vi "Convert to KRobot.vi"(10 "scale":dbl=1.0, 11 "Graphical Elements In":T2[](array[typedef])) -> (0 "Array":dbl[][][](array[numeric]) format="%#_3g", 2 "Kinematic Robot":refnum<class "NI_Robotics_Serial Robot Arm.lvclass">, 3 "Graphical Elements In 2":T2[](array[typedef]))   [LabVIEW 2017, in "NI_Robotics_3DKinematics.lvlib"]
uses:
  <vilib>/robotics/Kinematics/Plotting/NI_Robotics_3DKinematics.lvlib
  <vilib>/robotics/Kinematics/Robot/NI_Robotics_Serial Robot Arm.lvclass
  <vilib>/robotics/Kinematics/Plotting/Tree Element.ctl
  <vilib>/robotics/Kinematics/Plotting/Element Type.ctl
  <vilib>/robotics/Kinematics/Plotting/Joint Type.ctl
  <vilib>/Analysis/Matrix/Datatypes/RealMatrix.ctl
  <vilib>/robotics/Kinematics/Link/Joint Type.ctl
  <vilib>/robotics/Kinematics/Link/NI_Robotics_Link.lvclass
  <vilib>/Analysis/_algsub.llb/Real Vector Norm.vi
  <vilib>/Analysis/baseanly.llb/Real A x B.vi
  <vilib>/Analysis/baseanly.llb/Outer Product.vi
  <vilib>/Analysis/baseanly.llb/Real Outer Product.vi
  <vilib>/robotics/Kinematics/Create Lie Group Matrix.vi
  <vilib>/Analysis/Matrix/Numeric/Conversions/Array To Matrix - RA2.vi
  <vilib>/Analysis/7linalg.llb/Solve Linear Equations (multiple right hand).vi
  <vilib>/Analysis/Matrix/Numeric/Add/Add.vi
  <vilib>/Analysis/Matrix/Numeric/Add/Add - RM,RM.vi
  <vilib>/Analysis/Matrix/Numeric/Multiply/Multiply.vi
  <vilib>/Analysis/Matrix/Numeric/Multiply/Multiply - R,RM.vi
  <vilib>/Analysis/Matrix/Numeric/Multiply/Multiply - RM,R.vi
  <vilib>/Analysis/7linalg.llb/Create Special Matrix.vi
  <vilib>/Analysis/7linalg.llb/Create Special Real Matrix.vi
  <vilib>/Utility/AngleManip/Degrees to Radians (Scalar DBL).vi
  <vilib>/robotics/Kinematics/NI_Kinematics.lvlib
  <vilib>/Analysis/Matrix/NI_Matrix.lvlib
  <vilib>/Analysis/NI_AALPro.lvlib
  <vilib>/Analysis/NI_AALBase.lvlib
  <vilib>/Utility/AngleManip/NI_AngleManipulation.lvlib
panel:
  out "Array 3":T1[](array[typedef])
  out "A x B":dbl[][][](array[numeric]) format="%#_3g"
  out "Array 2":dbl[][](array[numeric])
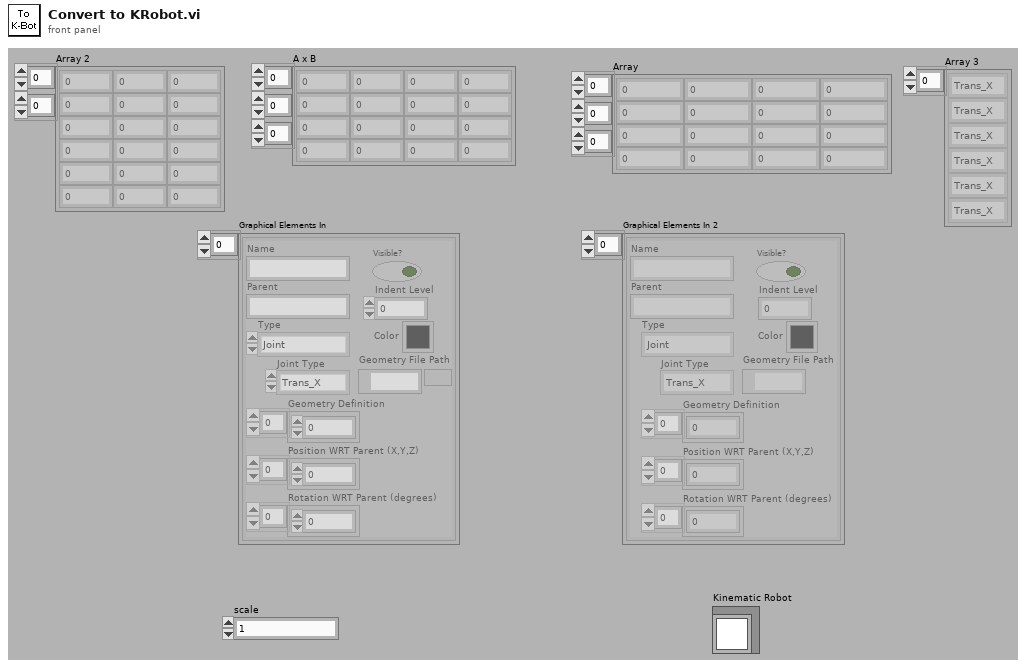
[diagram p1: front panel]
types:
  T1 = typedef "NI_Robotics_3DKinematics.lvlib/Joint Type.ctl" = enum16{"Trans_X", "Trans_Y", "Trans_Z", "Rot_X", "Rot_Y", "Rot_Z", "None"}
  T2 = typedef "NI_Robotics_3DKinematics.lvlib/Tree Element.ctl" = cluster{"Name":string, "Parent":string, "Type":T3, "Visible?":bool, "Geometry Definition":dbl[], "Position WRT Parent (X,Y,Z)":dbl[], "Rotation WRT Parent (degrees)":dbl[], "Joint Type":T1, "Geometry File Path":path, "Indent Level":i32, "Color":u32}
  T3 = typedef "NI_Robotics_3DKinematics.lvlib/Element Type.ctl" = enum16{"Joint", "Box", "Cylinder", "Cone", "Sphere", "ASE File", "VRML File", "STL File", "Space"}
  T4 = typedef "NI_Matrix.lvlib/RealMatrix.ctl" = dbl[][]
  T5 = typedef "NI_Robotics_Link.lvclass/Joint Type.ctl" = enum16{"Revolute", "Prismatic"}
  T6 = cluster{"Twist Angle":dbl, "Length":dbl, "Rotation Angle":dbl, "Offset Distance":dbl, "Joint Type":T5, "Joint Coordinate Offset":dbl}
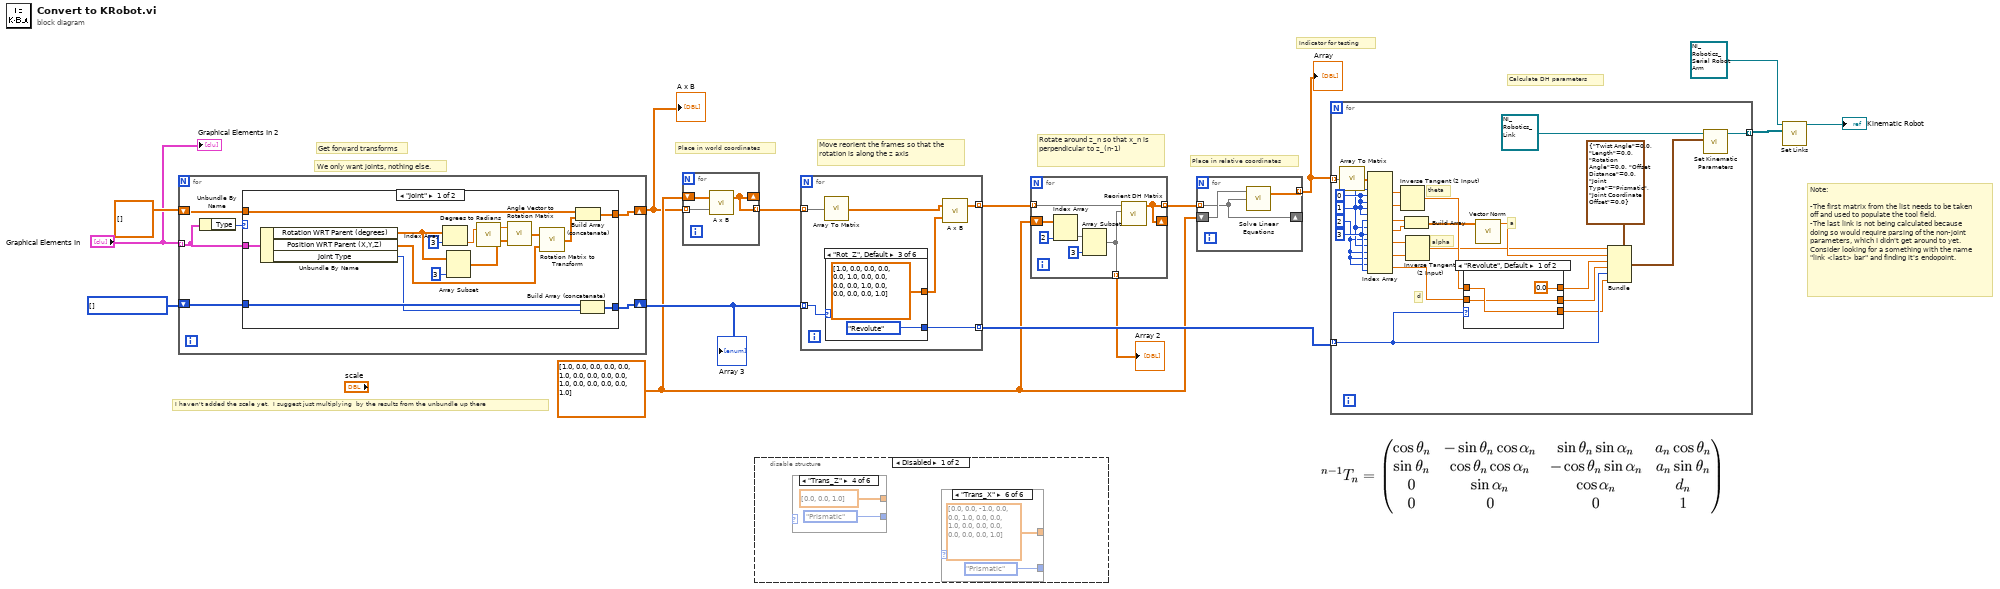
[diagram p0: block diagram]
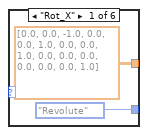
[diagram p2: hidden frame]
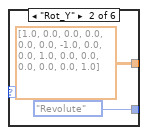
[diagram p3: hidden frame]
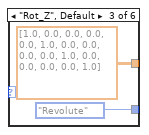
[diagram p4: hidden frame]
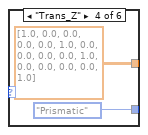
[diagram p5: hidden frame]
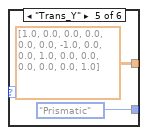
[diagram p6: hidden frame]
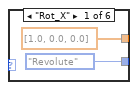
[diagram p7: hidden frame]
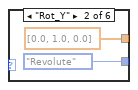
[diagram p8: hidden frame]
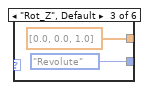
[diagram p9: hidden frame]
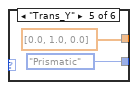
[diagram p10: hidden frame]
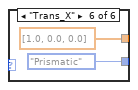
[diagram p11: hidden frame]
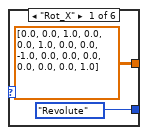
[diagram p13: hidden frame]
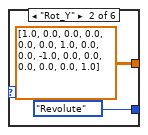
[diagram p14: hidden frame]
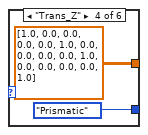
[diagram p15: hidden frame]
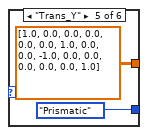
[diagram p16: hidden frame]
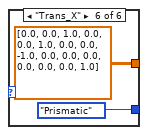
[diagram p17: hidden frame]
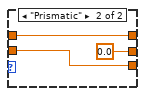
[diagram p18: hidden frame]
diagram:
  w10 = T1[] [] items=["Trans_X", "Trans_Y", "Trans_Z", "Rot_X", "Rot_Y", "Rot_Z", "None"]
  w6 = T4 [[1.0, 0.0, 0.0, 0.0], [0.0, 1.0, 0.0, 0.0], [0.0, 0.0, 1.0, 0.0], [0.0, 0.0, 0.0, 1.0]] ("Transform")
  # "I haven't added the scale yet.  I suggest just multiplying  by the results from the unbundle up there"
  # "Indicator for testing"
  # "Note:\n\n-The first matrix from the list needs to be taken off and used to populate the tool field.\n-The last link is not being calculated because doing so would require parsing of the non-joint parameters, which I didn't get around to yet.  Consider looking for a something with the name \"link <last> bar\" and finding it's endopoint."
  # "We only want joints, nothing else."
  # "Move reorient the frames so that the rotation is along the z axis"
  # "Place in relative coordinates"
  # "Rotate around z_n so that x_n is perpendicular to z_(n-1)"
  # "Place in world coordinates"
  # "Get forward transforms"
  # "Calculate DH parameters"
  n1 = for {
    tunnel: "Graphical Elements In" -> [w18] mode=indexing
    shift-right: [w19] -> w1
    shift-left: dbl[][][] [] -> [w20]
    shift-right: [w17] -> w9
    shift-left: w10 -> [w16]
    n2 = Unbundle By Name(w18) -> ("Type"=w21:T3)
    n3 = case shown="\"Joint\"" w21 {
      tunnel: w20 -> [w35 w38]
      tunnel: [w36 w38] -> w19
      tunnel: w18 -> [w34 _]
      tunnel: [w28 w37] -> w17
      tunnel: w16 -> [w29 w37]
      frame "Joint" {
        n4 = Unbundle By Name(w34) -> ("Rotation WRT Parent (degrees)"=w31:dbl[], "Position WRT Parent (X,Y,Z)"=w24:dbl[], "Joint Type"=w26:T1)
        n5 = Index Array(array=w31, index=3) -> (element=w23:dbl)
        n6 = Array Subset(array=w31, length=3) -> (w30:dbl[])  [unwired: 1 in]
        n7 = call-poly <vilib>:"Degrees to Radians.vi"("angle (deg)"=w23) -> ("angle (rad)"=w22:dbl)  [unwired: 2 in]
        n8 = call <vilib>:"Angle Vector to Rotation Matrix.vi"("vector"=w30, "angle"=w22) -> ("rotation matrix"=w27:T4)
        n9 = call <vilib>:"Rotation Matrix to Transform.vi"("translation vector"=w24, "rotation matrix"=w27) -> ("transform"=w25:T4)
        n10 = Build Array (concatenate)(w35, w25) -> (w36:dbl[][][])
        n11 = Build Array (concatenate)(w29, w26) -> (w28:T1[])
      }
      frame Default {
      }
    }
  }
  "A x B" <- w1
  "Array 3" <- w9
  n12 = for {
    tunnel: w1 -> [w40] mode=indexing
    shift-right: [w41] -> _
    shift-left: w6 -> [w39]
    tunnel: [w41] -> w7 mode=indexing
    n13 = call-poly <vilib>:"A x B.vi"("B"=w40, "A"=w39) -> ("A x B"=w41:T4)  [unwired: 1 out]
  }
  n14 = disable-structure shown="Disabled" {
    frame Disabled {
      n15 = case shown="\"Trans_Z\"" {
        selector: _ -> [_ _ _ _ _ _]
        tunnel: [dbl[] [1.0, 0.0, 0.0] dbl[] [0.0, 1.0, 0.0] dbl[] [0.0, 0.0, 1.0] dbl[] [0.0, 0.0, 1.0] dbl[] [0.0, 1.0, 0.0] dbl[] [1.0, 0.0, 0.0]] -> _
        tunnel: [Joint_Type."Revolute" ("Joint Type") Joint_Type."Revolute" ("Joint Type") Joint_Type."Revolute" ("Joint Type") Joint_Type."Prismatic" ("Joint Type") Joint_Type."Prismatic" ("Joint Type") Joint_Type."Prismatic" ("Joint Type")] -> _
        frame "Rot_X" {
        }
        frame "Rot_Y" {
        }
        frame "Rot_Z", Default {
        }
        frame "Trans_Z" {
        }
        frame "Trans_Y" {
        }
        frame "Trans_X" {
        }
      }
      n16 = case shown="\"Trans_X\"" {
        selector: _ -> [_ _ _ _ _ _]
        tunnel: [dbl[][] [[0.0, 0.0, -1.0, 0.0], [0.0, 1.0, 0.0, 0.0], [1.0, 0.0, 0.0, 0.0], [0.0, 0.0, 0.0, 1.0]] dbl[][] [[1.0, 0.0, 0.0, 0.0], [0.0, 0.0, -1.0, 0.0], [0.0, 1.0, 0.0, 0.0], [0.0, 0.0, 0.0, 1.0]] dbl[][] [[1.0, 0.0, 0.0, 0.0], [0.0, 1.0, 0.0, 0.0], [0.0, 0.0, 1.0, 0.0], [0.0, 0.0, 0.0, 1.0]] dbl[][] [[1.0, 0.0, 0.0, 0.0], [0.0, 1.0, 0.0, 0.0], [0.0, 0.0, 1.0, 0.0], [0.0, 0.0, 0.0, 1.0]] dbl[][] [[1.0, 0.0, 0.0, 0.0], [0.0, 0.0, -1.0, 0.0], [0.0, 1.0, 0.0, 0.0], [0.0, 0.0, 0.0, 1.0]] dbl[][] [[0.0, 0.0, -1.0, 0.0], [0.0, 1.0, 0.0, 0.0], [1.0, 0.0, 0.0, 0.0], [0.0, 0.0, 0.0, 1.0]]] -> _
        tunnel: [Joint_Type."Revolute" ("Joint Type") Joint_Type."Revolute" ("Joint Type") Joint_Type."Revolute" ("Joint Type") Joint_Type."Prismatic" ("Joint Type") Joint_Type."Prismatic" ("Joint Type") Joint_Type."Prismatic" ("Joint Type")] -> _
        frame "Rot_X" {
        }
        frame "Rot_Y" {
        }
        frame "Rot_Z", Default {
        }
        frame "Trans_Z" {
        }
        frame "Trans_Y" {
        }
        frame "Trans_X" {
        }
      }
    }
    frame Enabled {
    }
  }
  n17 = for {
    tunnel: w7 -> [w71] mode=indexing
    tunnel: w9 -> [w70] mode=indexing
    tunnel: [w69] -> w8 mode=indexing
    tunnel: [w68] -> w3 mode=indexing
    n18 = call-poly <vilib>:"Array To Matrix.vi"("Real 2D Array"=w71) -> ("Real Matrix"=w66:T4)
    n19 = case shown="\"Rot_Z\", Default" w70 {
      tunnel: [dbl[][] [[0.0, 0.0, 1.0, 0.0], [0.0, 1.0, 0.0, 0.0], [-1.0, 0.0, 0.0, 0.0], [0.0, 0.0, 0.0, 1.0]] dbl[][] [[1.0, 0.0, 0.0, 0.0], [0.0, 0.0, 1.0, 0.0], [0.0, -1.0, 0.0, 0.0], [0.0, 0.0, 0.0, 1.0]] dbl[][] [[1.0, 0.0, 0.0, 0.0], [0.0, 1.0, 0.0, 0.0], [0.0, 0.0, 1.0, 0.0], [0.0, 0.0, 0.0, 1.0]] dbl[][] [[1.0, 0.0, 0.0, 0.0], [0.0, 1.0, 0.0, 0.0], [0.0, 0.0, 1.0, 0.0], [0.0, 0.0, 0.0, 1.0]] dbl[][] [[1.0, 0.0, 0.0, 0.0], [0.0, 0.0, 1.0, 0.0], [0.0, -1.0, 0.0, 0.0], [0.0, 0.0, 0.0, 1.0]] dbl[][] [[0.0, 0.0, 1.0, 0.0], [0.0, 1.0, 0.0, 0.0], [-1.0, 0.0, 0.0, 0.0], [0.0, 0.0, 0.0, 1.0]]] -> w67
      tunnel: [Joint_Type."Revolute" ("Joint Type") Joint_Type."Revolute" ("Joint Type") Joint_Type."Revolute" ("Joint Type") Joint_Type."Prismatic" ("Joint Type") Joint_Type."Prismatic" ("Joint Type") Joint_Type."Prismatic" ("Joint Type")] -> w69
      frame "Rot_X" {
      }
      frame "Rot_Y" {
      }
      frame "Rot_Z", Default {
      }
      frame "Trans_Z" {
      }
      frame "Trans_Y" {
      }
      frame "Trans_X" {
      }
    }
    n20 = call-poly <vilib>:"A x B.vi"("B"=w67, "A"=w66) -> ("A x B"=w68:T4)  [unwired: 1 out]
  }
  n21 = for {
    shift-right: [w87] -> _
    shift-left: w6 -> [w85]
    tunnel: [w87] -> w5 mode=indexing
    tunnel: w3 -> [w86] mode=indexing
    tunnel: [w84] -> w4 mode=indexing
    n22 = Index Array(array=w85, index (col)=2) -> (element=w90:dbl[])  [unwired: 1 in]
    n23 = Array Subset(array=w90, length=3) -> (w84:dbl[])  [unwired: 1 in]
    n24 = call <vilib>:"Reorient DH Matrix.vi"("z"=w84, "Original Frame"=w86) -> ("Reoriented Frame"=w87:T4)  [unwired: 9 in]
  }
  "Array 2" <- w4
  n25 = for {
    shift-right: [w91] -> _
    shift-left: w6 -> [w93]
    tunnel: [w92] -> w2 mode=indexing
    tunnel: w5 -> [w91] mode=indexing
    n26 = call-poly <vilib>:"Solve Linear Equations.vi"("Known Matrix"=w91, "Input Matrix"=w93) -> ("Solution Matrix"=w92:T4)  [unwired: 1 in, 1 out]
  }
  "Array" <- w2
  n27 = for {
    tunnel: w2 -> [w95] mode=indexing
    tunnel: [w117] -> w15 mode=indexing
    tunnel: w8 -> [w114] mode=indexing
    w94 = 2 ("index (row)")
    w100 = 3 ("index (row)")
    w97 = 1 ("index (row)")
    w107 = 0 ("index (col)")
    # "alpha"
    # "a"
    # "d"
    # "theta"
    n28 = call-poly <vilib>:"Array To Matrix.vi"("Real 2D Array"=w95) -> ("Real Matrix"=w96:T4)
    n29 = Index Array(array=w96, index (row) #1=w97, index (col) #1=w107, index (row) #2=w107, index (col) #2=w107, index (row) #3=w107, index (col) #3=w100, index (row) #4=w97, index (col) #4=w100, index (row) #5=w94, index (col) #5=w97, index (row) #6=w94, index (col) #6=w94, index (row) #7=w94, index (col) #7=w100) -> (element #1=w109:dbl, element #2=w110:dbl, element #3=w106:dbl, element #4=w105:dbl, element #5=w102:dbl, element #6=w101:dbl, element #7=w99:dbl)
    n30 = Inverse Tangent (2 Input)(1:w110, 2:w109) -> (0:w108:dbl)
    n31 = Build Array(w106, w105) -> (w104:dbl[])
    n32 = Inverse Tangent (2 Input)(1:w101, 2:w102) -> (0:w98:dbl)
    n33 = case shown="\"Revolute\", Default" w114 {
      tunnel: [w120 w122] -> w113
      tunnel: [w119 0.0] -> w112
      tunnel: [0.0 w123] -> w111
      tunnel: w108 -> [w120 w123]
      tunnel: w99 -> [w119 w122]
      frame "Revolute", Default {
      }
      frame "Prismatic" {
      }
    }
    n34 = call-poly <vilib>:"Vector Norm.vi"("Input Vector"=w104) -> ("norm"=w103:dbl)  [unwired: 9 in, 1 out]
    n35 = Bundle(cluster=T6 {"Twist Angle"=0.0, "Length"=0.0, "Rotation Angle"=0.0, "Offset Distance"=0.0, "Joint Type"=enum."Prismatic", "Joint Coordinate Offset"=0.0} ("Parameters"), "Twist Angle"=w98, "Length"=w103, "Rotation Angle"=w111, "Offset Distance"=w112, "Joint Type"=w114, "Joint Coordinate Offset"=w113) -> (w116:T6)
    n36 = call <vilib>:"Set Kinematic Parameters.vi"("kinematic parameters"=w116, "link in"=refnum<class "NI_Robotics_Link.lvclass"> refnum ("Link")) -> ("link out"=w117:refnum<class "NI_Robotics_Link.lvclass">)  [unwired: 8 in, 1 out]
  }
  n37 = call <vilib>:"Set Links.vi"("links"=w15, "serial arm in"=refnum<class "NI_Robotics_Serial Robot Arm.lvclass"> refnum ("Robot.lvclass")) -> ("serial arm out"=→"Kinematic Robot":refnum<class "NI_Robotics_Serial Robot Arm.lvclass">)  [unwired: 8 in, 1 out]
  "Graphical Elements In 2" <- "Graphical Elements In"
